vi "Test_WriteNewItem_NotReplaced.vi"(8 "error in (no error)":errorcluster, 11 "TestCase in":refnum<class "TestComposedLookupTable.lvclass">) -> (0 "error out":errorcluster, 3 "TestCase out":refnum<class "TestComposedLookupTable.lvclass">)   [LabVIEW 2017, in "TestComposedLookupTable.lvclass"]
uses:
  TestComposedLookupTable.lvclass
  Source/LookupTable/LookupTable.lvclass/LookupTable.ctl
  da2d8a2f-264c-46cc-987c-9c5462641e62.vi
  Source/LookupTable/Read Table Reference.vi
  da2d8a2f-264c-46cc-987c-9c5462641e62.vi/2f0e9c6e-b231-4656-b7f8-361b1a7b5d67.vi
  Source/LookupTable/LookupTable.lvclass
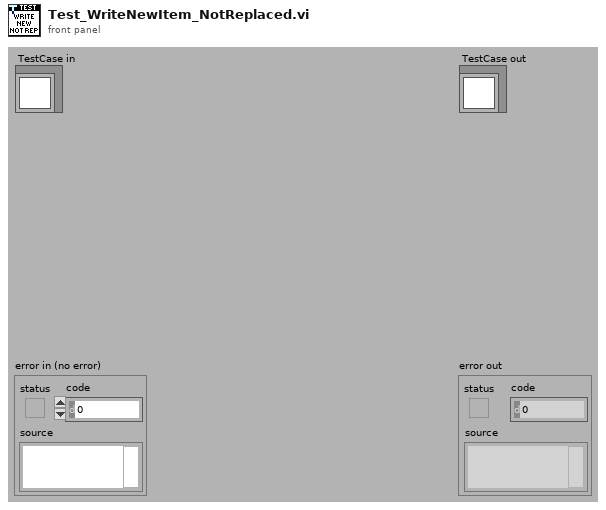
[diagram p1: front panel]
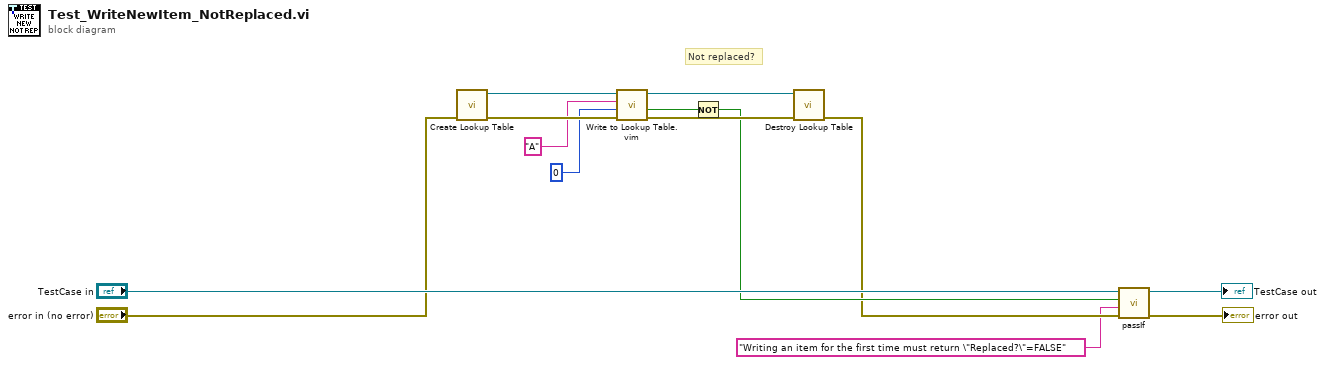
[diagram p0: block diagram]
diagram:
  # "Not replaced?"
  n1 = call "Create Lookup Table.vi"("error in (no error)"="error in (no error)") -> ("error out"=w13:errorcluster, "LookupTable Reference"=w5:refnum<data-value>)  [unwired: 9 in]
  n2 = call "Write to Lookup Table.vim"("error in (no error)"=w13, "Item"=0, "Item Name"="A", "LookupTable Reference"=w5) -> ("error out"=w14:errorcluster, "Replaced?"=w7:bool, "LookupTable Reference Out"=w3:refnum<data-value>)  [unwired: 5 in]
  n3 = Not(x=w7) -> (.not. x?=w6:bool)
  n4 = call "Destroy Lookup Table.vi"("error in (no error)"=w14, "LookupTable Reference"=w3) -> ("error out"=w2:errorcluster)  [unwired: 9 in]
  n5 = call-dynamic "passIf.vi"("error in (no error)"=w2, "message (\"\")"="Writing an item for the first time must return \"Replaced?\"=FALSE" ("message (\"\")"), "pass"=w6, "TestCase in"="TestCase in") -> ("error out"=→"error out":errorcluster, "TestCase out"=→"TestCase out":refnum<class "TestComposedLookupTable.lvclass">)  [unwired: 6 in]
